vi "Verwaltung Stickstoff Befuellung.vi"(8 "Fehler (Eingang)":errorcluster) -> (0 "Fehler (Ausgang)":errorcluster)   [LabVIEW 2020, in "Stickstoff Befuellung.lvlib"]
uses:
  Stickstoff Befuellung.lvlib
  Konfig-Dateien/FGV Betriebsdaten Aktionen.ctl
  Aktionen Stockstoff Befuellung.ctl
  Verwaltung/FGV OUT Aktionen.ctl
  Allgemein/FGV FT-IR Kuehlung Aktionen.ctl
  Konfig-Dateien/Aktionen Konfig.ctl
  Konfig-Dateien/Konfig-Dateien.lvlib
  Verwaltung/Verwaltung - cRIO.lvlib
  Allgemein/Allgemein.lvlib
  Seiten/Log Konfig/Auswahlfeld aktiviert-deaktiviert.ctl
  Seiten/Log Konfig/LogKonfig.lvlib
panel:
  # "Verwaltung Stickstoff Befüllung"
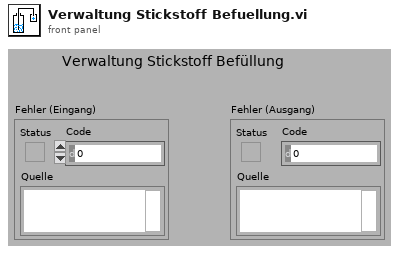
[diagram p1: front panel]
types:
  T1 = typedef "Konfig-Dateien.lvlib/FGV Betriebsdaten Aktionen.ctl" = enum16{"lesen", "Anlagengrenzw.", "PID Param.", "Sonstige", "Sensor Para."}
  T2 = typedef "Erweiterte Konfig.lvlib/Sonstige Parameter.ctl" = cluster{"Lüfter langsam":sgl, "Lüfter schnell":sgl, "FT-IR Kühlung Soll":sgl, "FT-IR Kühlung Max":sgl, "Überwachung":T3, "Befüllung aktiv":T4, "Stickstoff Befüllzeit":sgl, "Befüllintervall":sgl, "Kalibrierwert FT-IR":sgl, "Offset Ausgang":sgl, "Offset FT-IR":sgl, "Offset Druck FT-IR":sgl, "Dichtheitstest Zeit":sgl, "Dichtheitstest Abfall":sgl, "Dichtheitstest Umfang":T5, "Offset Umgebung":sgl, "Max Taupunkt":sgl, "Pumpendrehzahl":sgl, "ext. Befüllung":T4, "Ext. Stickstoff Befüllzeit":sgl}
  T3 = typedef "Auswahlfeld.ctl" = u16
  T4 = typedef "LogKonfig.lvlib/Auswahlfeld aktiviert-deaktiviert.ctl" = u16
  T5 = typedef "Erweiterte Konfig.lvlib/Dichtheitstest Umfang.ctl" = u16
  T6 = typedef "Allgemein.lvlib/FGV FT-IR Kuehlung Aktionen.ctl" = enum16{"lesen", "Kühlung?"}
  T7 = typedef "Verwaltung - cRIO.lvlib/FGV OUT Aktionen.ctl" = enum16{"lesen", "ANA OUT", "DO 0-31", "DO 32-47"}
  T8 = typedef "Stickstoff Befuellung.lvlib/Aktionen Stockstoff Befuellung.ctl" = enum16{"lesen", "Befüllen vorbereiten", "Befüllen", "Befüllen beenden", "Warten", "deaktiviert", "initialisieren", "anstehender Fehler"}
  T9 = typedef "Konfig-Dateien.lvlib/Aktionen Konfig.ctl" = enum16{"lesen", "laden", "speichern  System.ini", "speichern Anlagengrenzw.", "speichern PID + Sonstige", "speichern BSZ BMP", "speichern BSZ FT-IR", "speichern Stickstoff Bef.", "speichern Ext. Stickstoff Bef.", "speichern CAN_Konfig"}
  T10 = typedef "Verwaltung - cRIO.lvlib/Digital Ausgaenge 0-31.ctl" = cluster{"O0: Druckluft Versorgung":bool, "O1: CG 1 (FB Eingang 1)":bool, "O2: CG 2 (Kühlung FT-IR EIN)":bool, "O3: CG 3 (FB Bypass)":bool, "O4: CG 4 (FB CalGas)":bool, "O5: CG 5 (FB spülen/UL)":bool, "O6: CG 6 (FB zum FT-IR)":bool, "O7: CG 7 (FB zum FID)":bool, "O8: CG 8 (FB Reserve)":bool, "O9: (FB Reserve)":bool, "O10: (FB Umgebungsluft FID)":bool, "O11: (FB zum Gaskühler)":bool, "O12: FB Stickstoff zu FT-IR":bool, "O13: Optikbox FT-IR spülen":bool, "O14: (Purifier deaktivieren)":bool, "O15: (Umschaltung Purifier/Stickstoff)":bool, "O16: N2 Einblasung":bool, "O17: LSP LN2 Nachfüllung":bool, "O18: (Reserve)":bool, "O19: (Pumpe Eingang1)":bool, "O20: (Pumpe Eingang2)":bool, "O21: (Pumpe Spülen1)":bool, "O22: (Pumpe Spülen2)":bool, "O23: (Reserve)":bool, "O24: CalGas 1":bool, "O25: CalGas 2":bool, "O26: CG 3-8 (CalGas 3)":bool, "O27: Stickstoff aufschalten":bool, "O28: CG zu PNS":bool, "O29: FTIR Standby Spülung":bool, "O30: CG zu Entnahme(T90)":bool, "O31: (Purifier regenerieren)":bool}
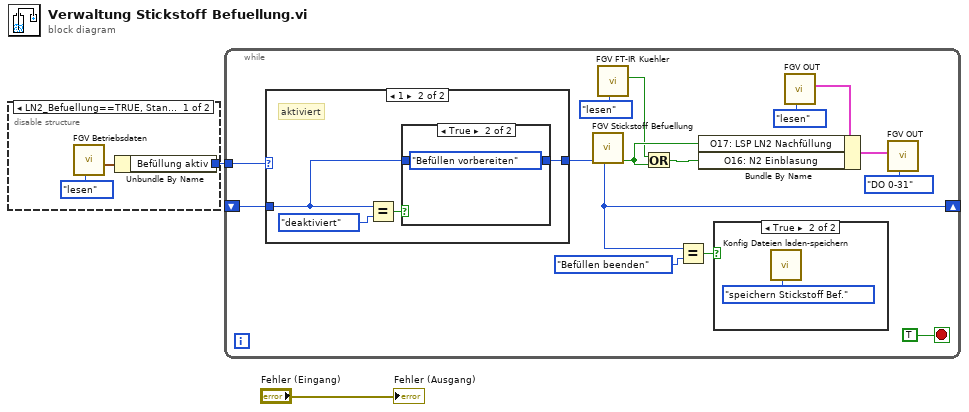
[diagram p0: block diagram]
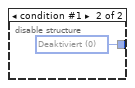
[diagram p2: hidden frame]
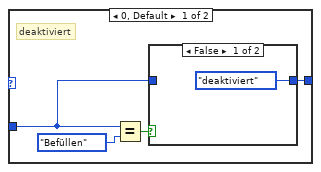
[diagram p4: hidden frame]
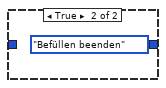
[diagram p5: hidden frame]
diagram:
  n1 = disable-structure shown="LN2_Befuellung==TRUE, Standard" {
    disable-tunnel: [w5 w6] -> w2
    frame condition #0 (active) {
      n2 = call "FGV Betriebsdaten.vi"("Aktionen"=FGV_Betriebsdaten_Aktionen."lesen") -> ("Sonstige"=w3:T2)  [unwired: 7 in, 3 out]
      n3 = Unbundle By Name(w3) -> ("Befüllung aktiv"=w5:T4)
    }
    frame condition #1 {
      w6 = T4 0 items=["Deaktiviert", "Aktiviert"] ("Befüllung aktiv")
    }
  }
  n4 = while {
    shift-right: [w16] -> _
    shift-left: _ -> [w20]
    tunnel: w2 -> [w18]
    stop <- TRUE stop-if-true
    n5 = case shown="1" w18 {
      tunnel: w20 -> [w24 w30]
      tunnel: [w23 w29] -> w19
      frame 0, Default {
        # "deaktiviert"
        n6 = Equal?(x=w24, y=Aktionen_Stockstoff_Befuellung."Befüllen" ("x")) -> (x = y?=w25:bool)
        n7 = case shown="False" w25 {
          tunnel: w24 -> [_ _]
          tunnel: [Aktionen_Stockstoff_Befuellung."deaktiviert" ("Aktion") Aktionen_Stockstoff_Befuellung."Befüllen beenden" ("Aktion")] -> w23
          frame False {
          }
          frame True {
          }
        }
      }
      frame 1 {
        # "aktiviert"
        n8 = Equal?(x=w30, y=Aktionen_Stockstoff_Befuellung."deaktiviert" ("x")) -> (x = y?=w31:bool)
        n9 = case shown="True" w31 {
          tunnel: w30 -> [w33 _]
          tunnel: [w33 Aktionen_Stockstoff_Befuellung."Befüllen vorbereiten" ("Aktion")] -> w29
          frame False {
          }
          frame True {
          }
        }
      }
    }
    n10 = call "FGV Stickstoff Befuellung.vi"("Aktion"=w19) -> ("Ausgang"=w9:bool, "Aktion"=w16:T8)  [unwired: 4 in, 5 out]
    n11 = call "FGV FT-IR Kuehler.vi"("Aktionen"=FGV_FT-IR_Kuehlung_Aktionen."lesen") -> ("LN2 Spülen"=w8:bool)  [unwired: 6 in, 4 out]
    n12 = Or(x=w8, y=w9) -> (x .or. y?=w7:bool)
    n13 = Equal?(x=w16, y=Aktionen_Stockstoff_Befuellung."Befüllen beenden" ("x")) -> (x = y?=w15:bool)
    n14 = case shown="True" w15 {
      frame False {
      }
      frame True {
        n15 = call "Konfig Dateien laden-speichern.vi"("Aktion"=Aktionen_Konfig."speichern Stickstoff Bef.") -> ()  [unwired: 10 in, 1 out]
      }
    }
    n16 = call "FGV OUT.vi"("Aktion"=FGV_OUT_Aktionen."lesen") -> ("DO 0-31"=w13:T10)  [unwired: 7 in, 3 out]
    n17 = Bundle By Name(cluster=w13, "O17: LSP LN2 Nachfüllung"=w9, "O16: N2 Einblasung"=w7) -> (w11:T10)
    n18 = call "FGV OUT.vi"("Aktion"=FGV_OUT_Aktionen."DO 0-31", "DO 0-31"=w11) -> ()  [unwired: 6 in, 4 out]
  }
  "Fehler (Ausgang)" <- "Fehler (Eingang)"
